vi "LUT - Test Empty.vi"(8 "error in (no error)":errorcluster) -> (0 "error out":errorcluster)   [LabVIEW 2017]
uses:
  <vilib>/addons/_JKI Toolkits/Caraya/classes/Assert/Assert True.vi
  <vilib>/addons/_JKI Toolkits/Caraya/classes/Assert/Assert False.vi
  <vilib>/addons/_JKI Toolkits/Caraya/classes/Test/Test.lvclass
  src/LUT/LUT.lvclass
  <vilib>/addons/_JKI Toolkits/Caraya/classes/Assert/Assert.lvclass
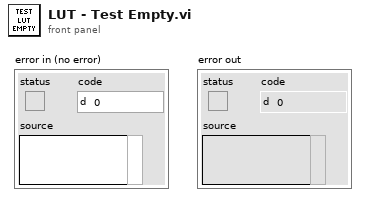
[diagram p1: front panel]
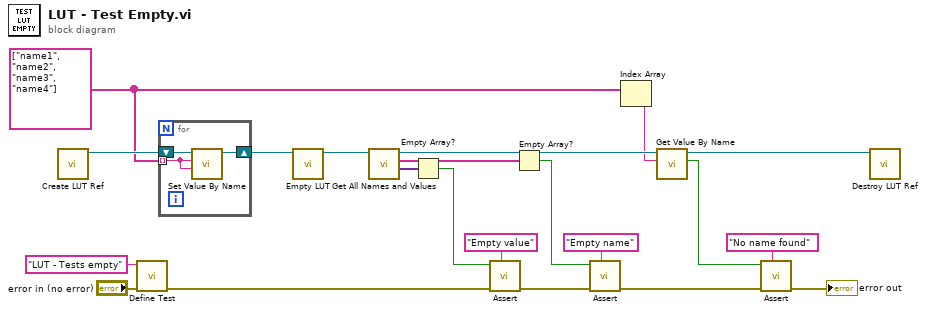
[diagram p0: block diagram]
diagram:
  w6 = string[] ["name1", "name2", "name3", "name4"]
  n1 = call "Create LUT Ref.vi"() -> ("LUT out"=w15:refnum<class "LUT.lvclass">)  [unwired: 10 in, 1 out]
  n2 = call <vilib>:"Define Test.vi"("error in (no error)"="error in (no error)", "Label (VI Title)"="LUT - Tests empty") -> ("error out"=w12:errorcluster)  [unwired: 9 in]
  n3 = for {
    shift-right: [w23] -> w14
    shift-left: w15 -> [w24]
    tunnel: w6 -> [w22] mode=indexing
    n4 = call "Set Value By Name.vi"("Value"=w22, "Name"=w22, "LUT in"=w24) -> ("LUT out"=w23:refnum<class "LUT.lvclass">)  [unwired: 6 in, 2 out]
  }
  n5 = call "Empty LUT.vi"("LUT in"=w14) -> ("LUT out"=w13:refnum<class "LUT.lvclass">)  [unwired: 9 in, 1 out]
  n6 = call "Get All Names and Values.vi"("LUT in"=w13) -> ("Values"=w11:variant[], "Names"=w9:string[], "LUT out"=w16:refnum<class "LUT.lvclass">)  [unwired: 7 in, 1 out]
  n7 = Empty Array?(array=w11) -> (empty?=w10:bool)
  n8 = call-poly <vilib>:"Assert.vi"("Label"="Empty value", "error in (no error)"=w12, "True?"=w10) -> ("error out"=w18:errorcluster)  [unwired: 8 in]
  n9 = Empty Array?(array=w9) -> (empty?=w8:bool)
  n10 = call-poly <vilib>:"Assert.vi"("Label"="Empty name", "error in (no error)"=w18, "True?"=w8) -> ("error out"=w4:errorcluster)  [unwired: 8 in]
  n11 = Index Array(array=w6) -> (element=w5:string)  [unwired: 1 in]
  n12 = call "Get Value By Name.vi"("Name"=w5, "LUT in"=w16) -> ("found?"=w1:bool, "LUT out"=w7:refnum<class "LUT.lvclass">)  [unwired: 6 in, 2 out]
  n13 = call-poly <vilib>:"Assert.vi"("Label"="No name found", "error in (no error)"=w4, "False?"=w1) -> ("error out"=→"error out":errorcluster)  [unwired: 8 in]
  n14 = call "Destroy LUT Ref.vi"("LUT in"=w7) -> ()  [unwired: 10 in, 1 out]
